vi "Property Node (Hardware).vi"   [LabVIEW 2012, in "nisyscfg.lvlib"]
doc: "Gets (reads) and/or sets (writes) properties for system hardware. Wire the Save Changes VI to the property node after you have finished setting all the properties.\n\nRefer to Property Node (Hardware) Descriptions for descriptions of the available properties."
uses:
  <vilib>/nisyscfg/nisyscfg.lvlib
  <resource>/objmgr/nisysapi.rc
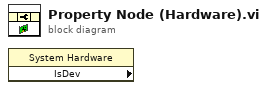
[diagram p0: block diagram]
diagram:
  n1 = property class="System Hardware" props=["IsDev"]() -> ()  [unwired: 2 in, 3 out]
